vi "CBSControlling.vi"() -> ()   [LabVIEW 2015]
uses:
  classes/DataHandlerMYiTOPS.lvclass
panel:
  in  "Monitoring":T1 {"Meter" scale=0.0..20.0}
  out "appended array":string[](array[string])
  out "element":string
  out "Control-Matrix-Overview 2":i32(listbox)=-1
  in  "Controlling":T2
  in  "Cyber-physical Objects":i32(listbox)
  in  "Stop":bool
  out "Control-Matrix-Overview":i32(listbox)=-1
  # "Hard Key:"
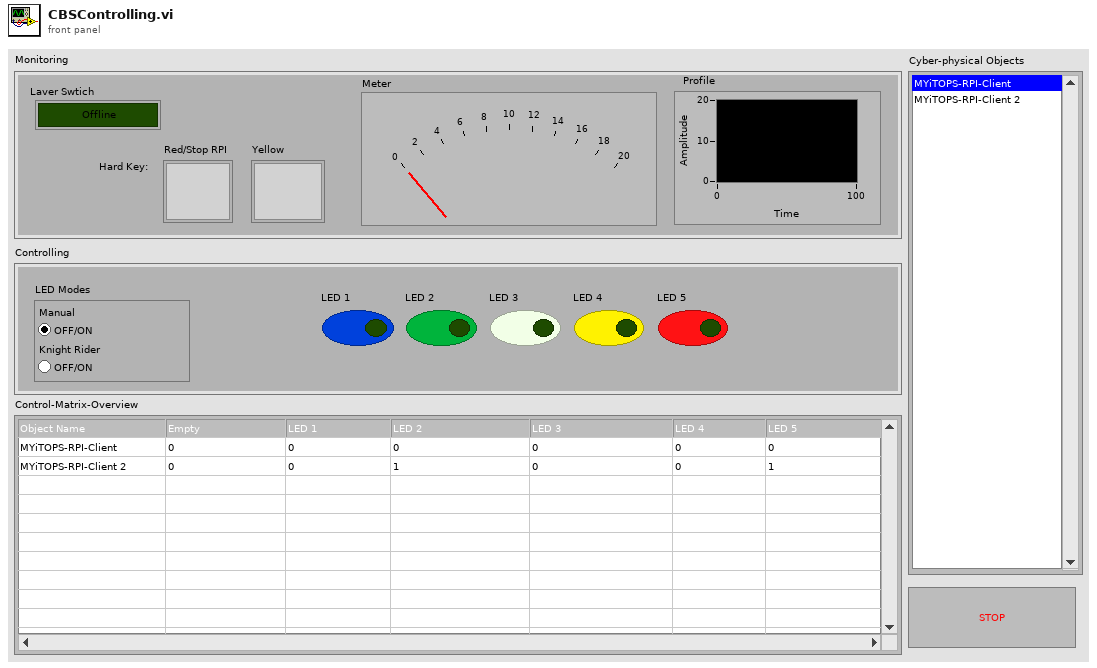
[diagram p1: front panel]
types:
  T1 = cluster{"Meter":i8, "Profile":dbl, "Yellow":bool, "Red/Stop RPI":bool, "Laver Swtich":bool}
  T2 = cluster{"LED 1":bool, "LED 5":bool, "LED 2":bool, "LED 3":bool, "LED 4":bool, "LED Modes":enum32{"Manual", "Knight Rider"}}
  T3 = enum8{"Enabled", "Disabled", "Disabled and Grayed Out"}
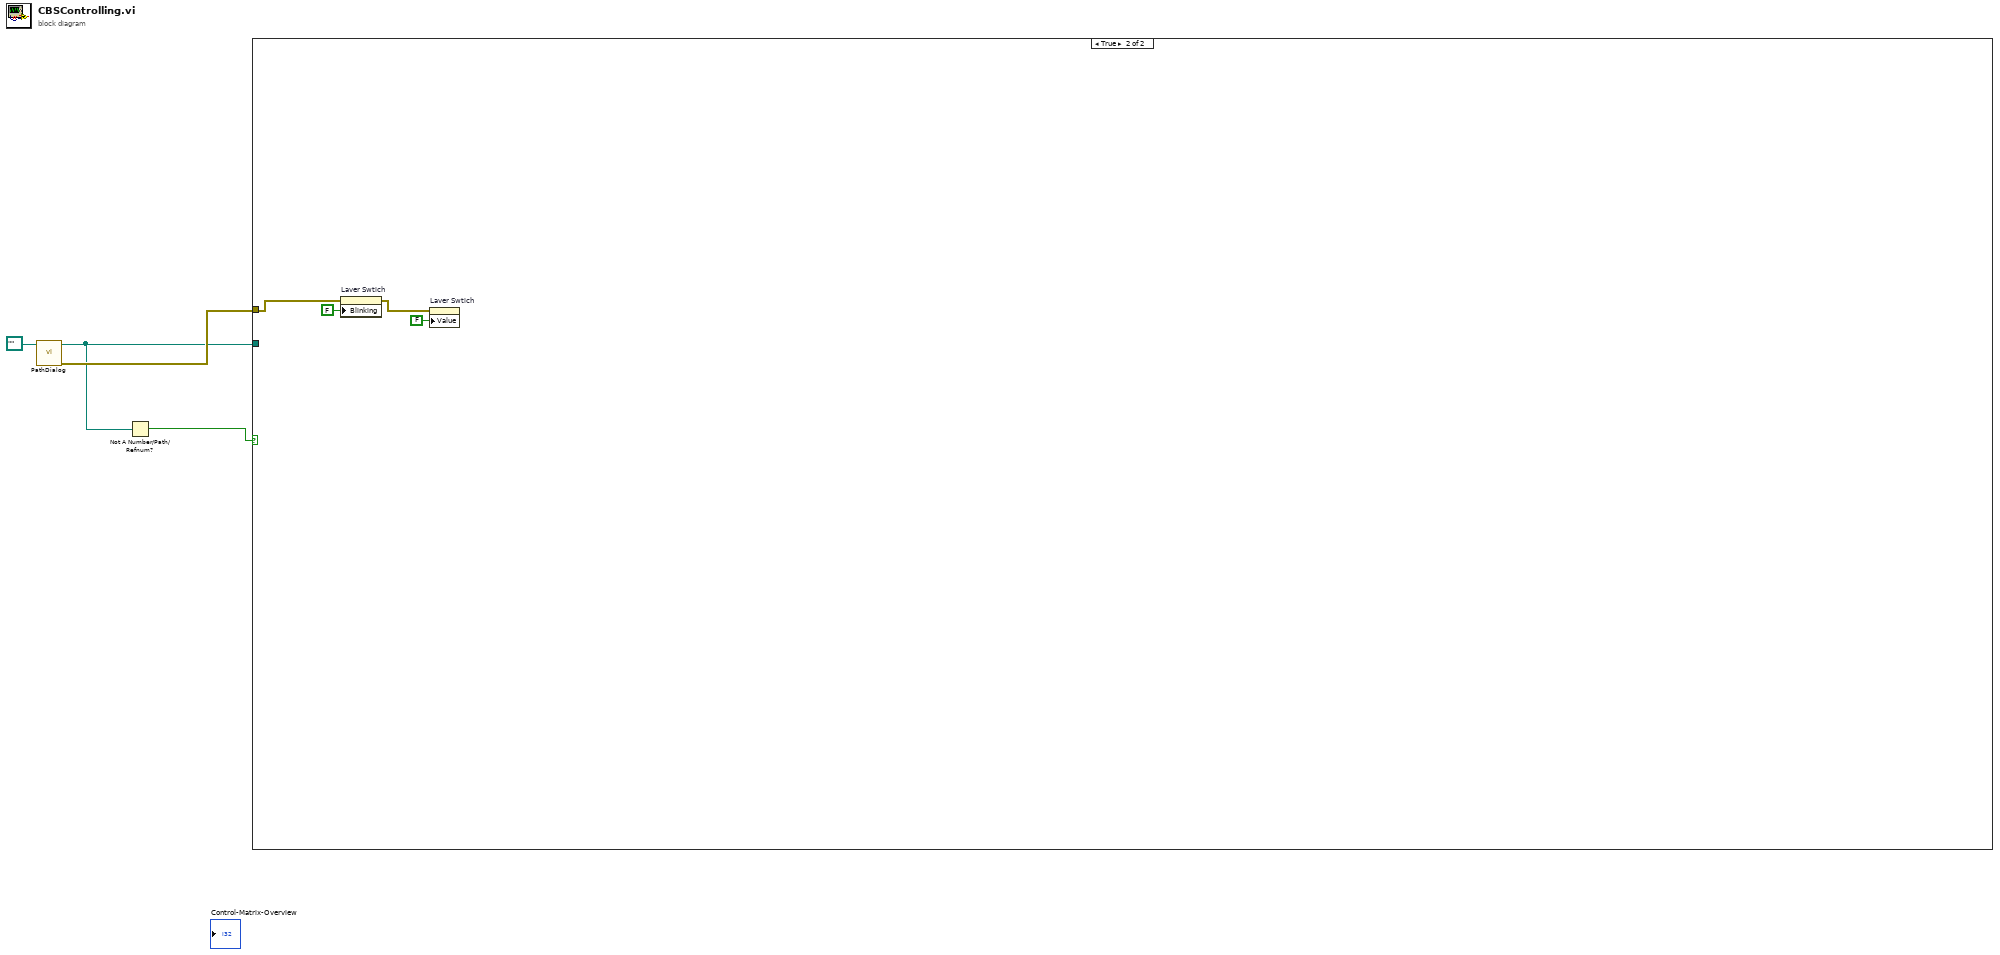
[diagram p0: block diagram]
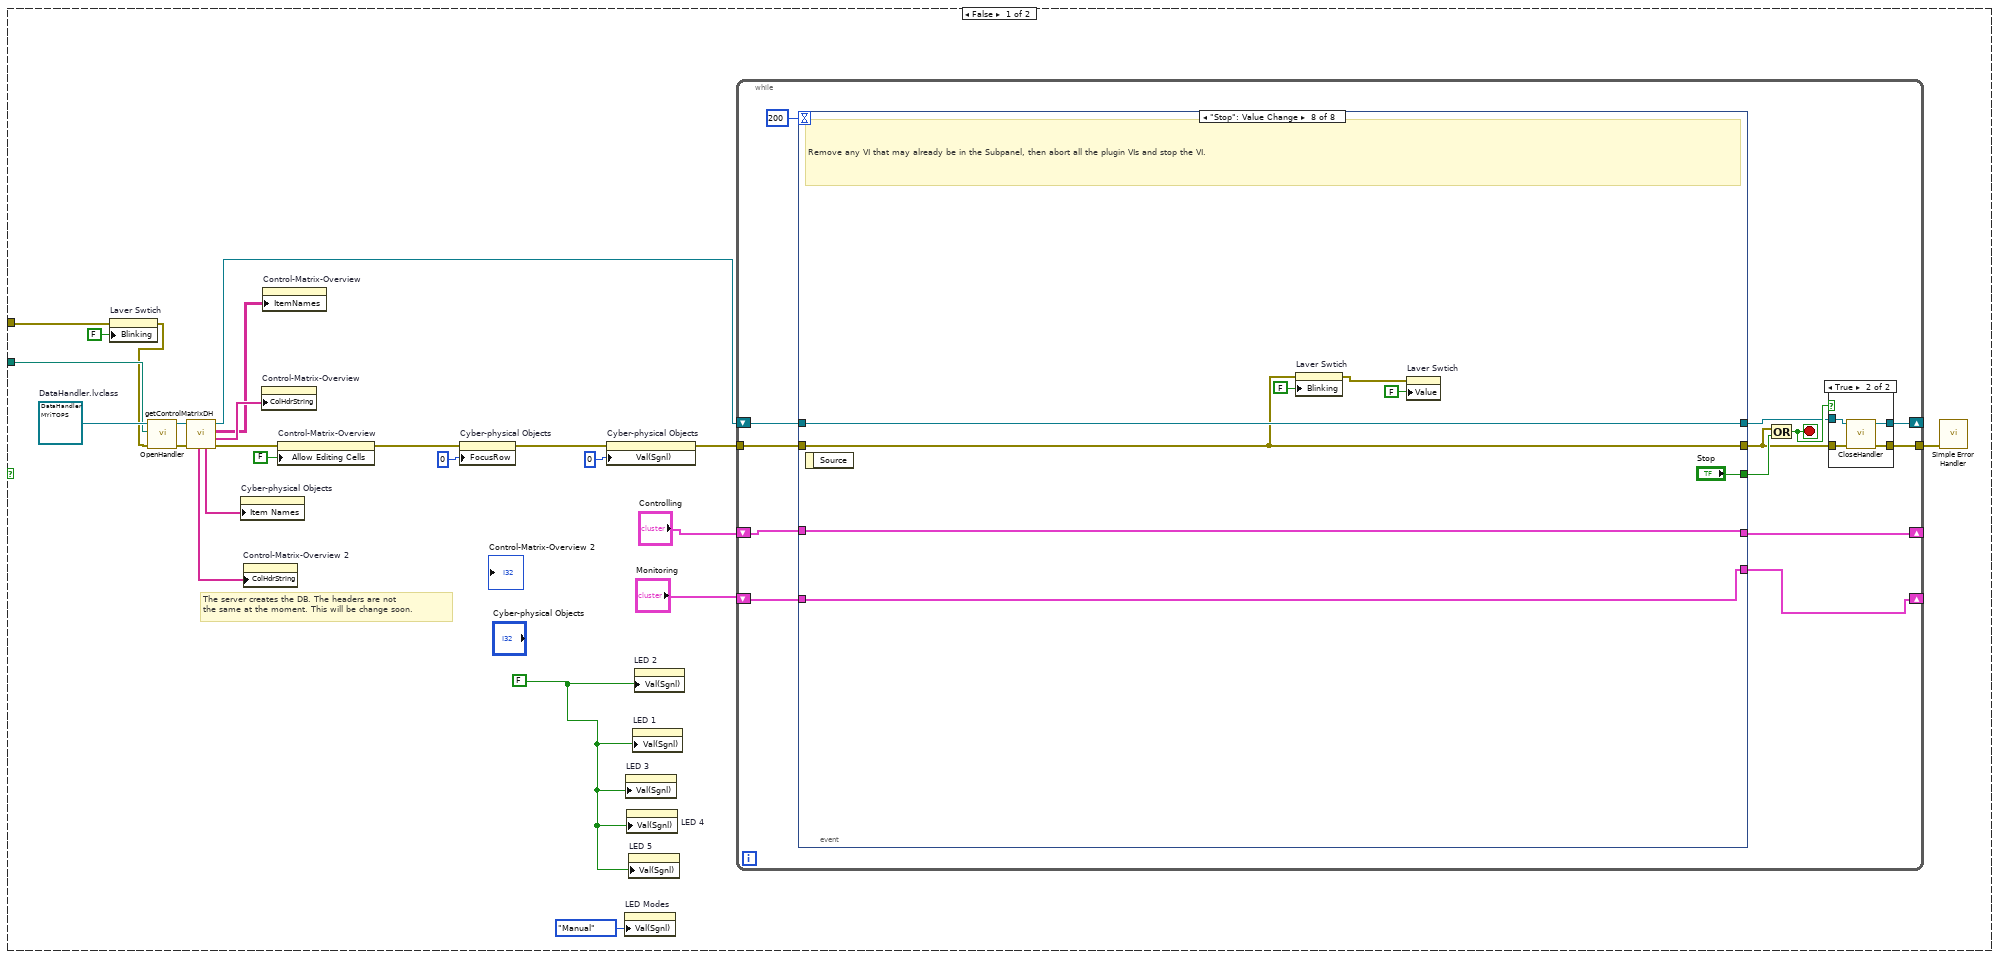
[diagram p2: hidden frame]
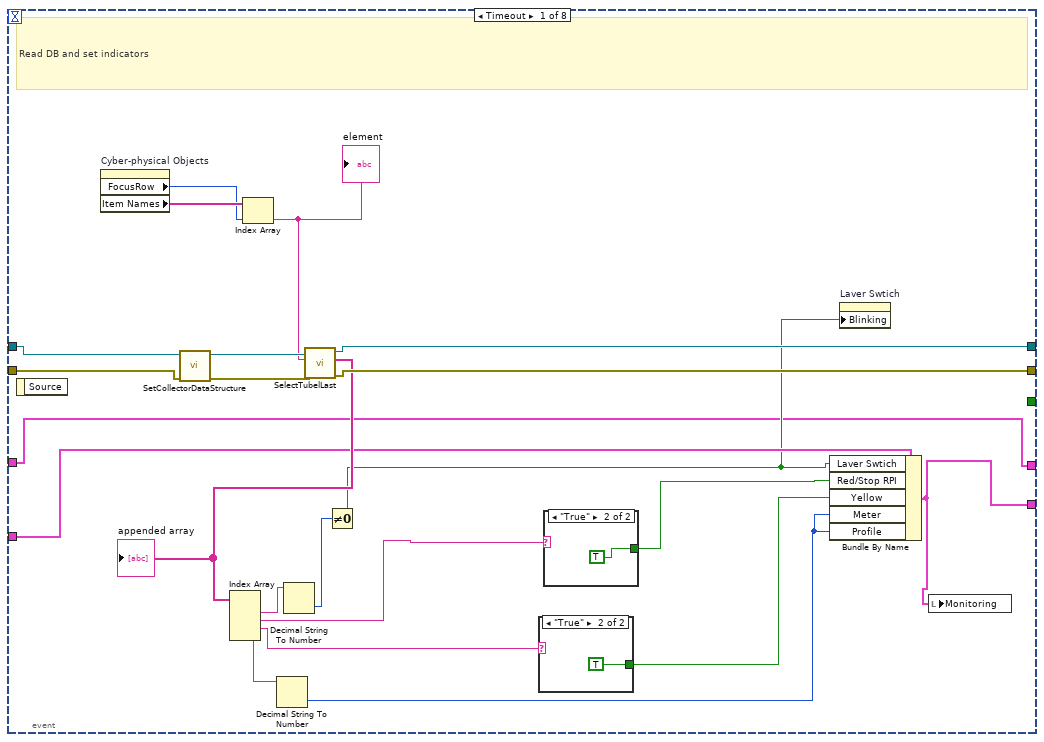
[diagram p4: hidden frame]
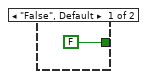
[diagram p5: hidden frame]
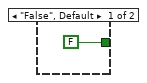
[diagram p6: hidden frame]
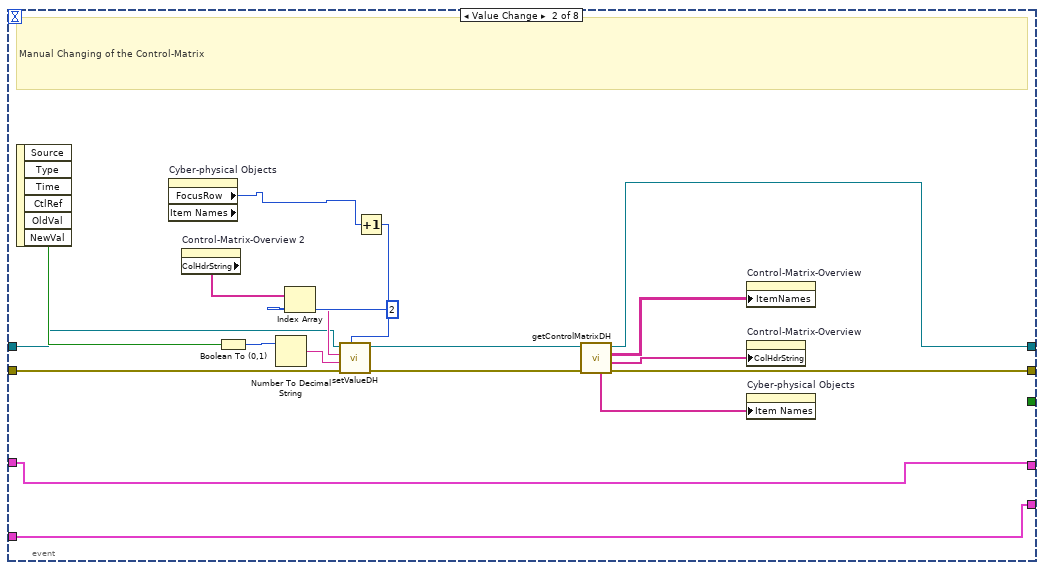
[diagram p7: hidden frame]
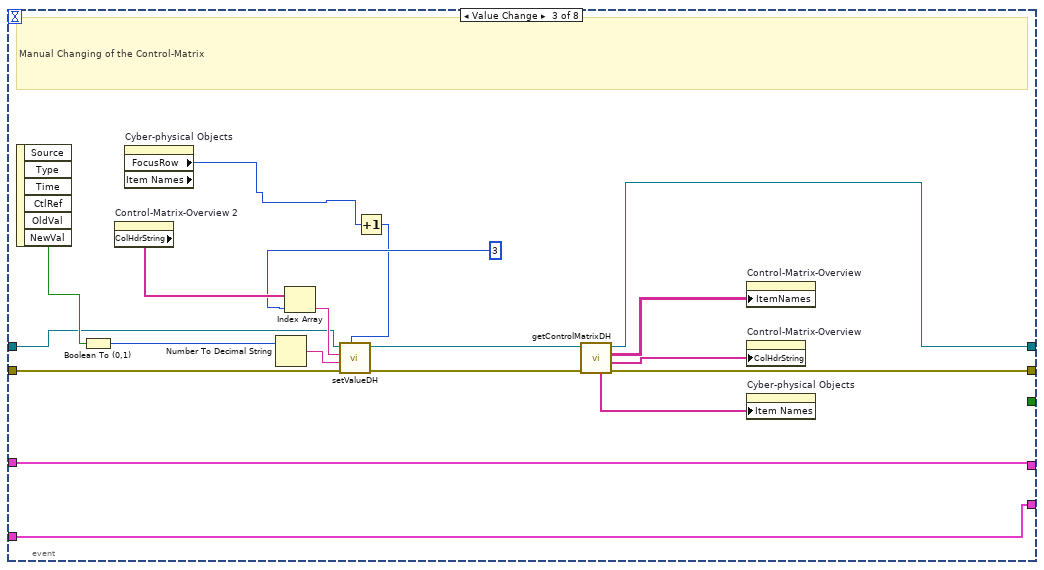
[diagram p8: hidden frame]
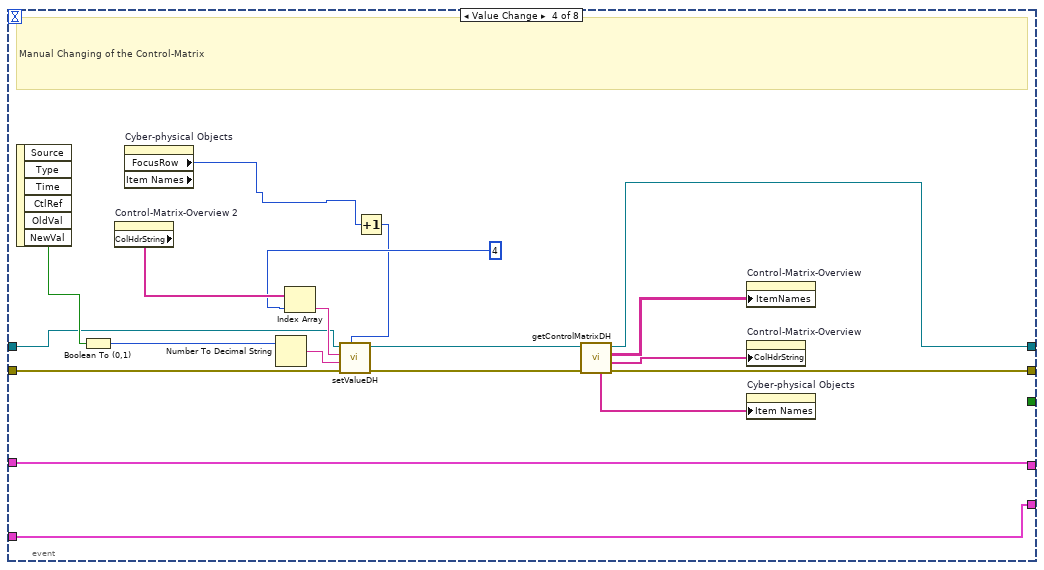
[diagram p9: hidden frame]
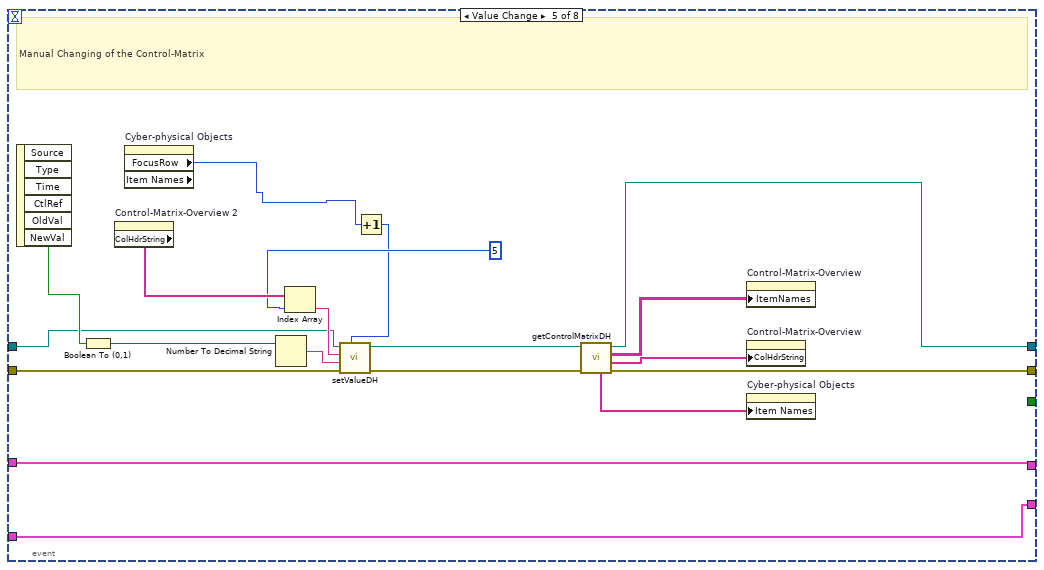
[diagram p10: hidden frame]
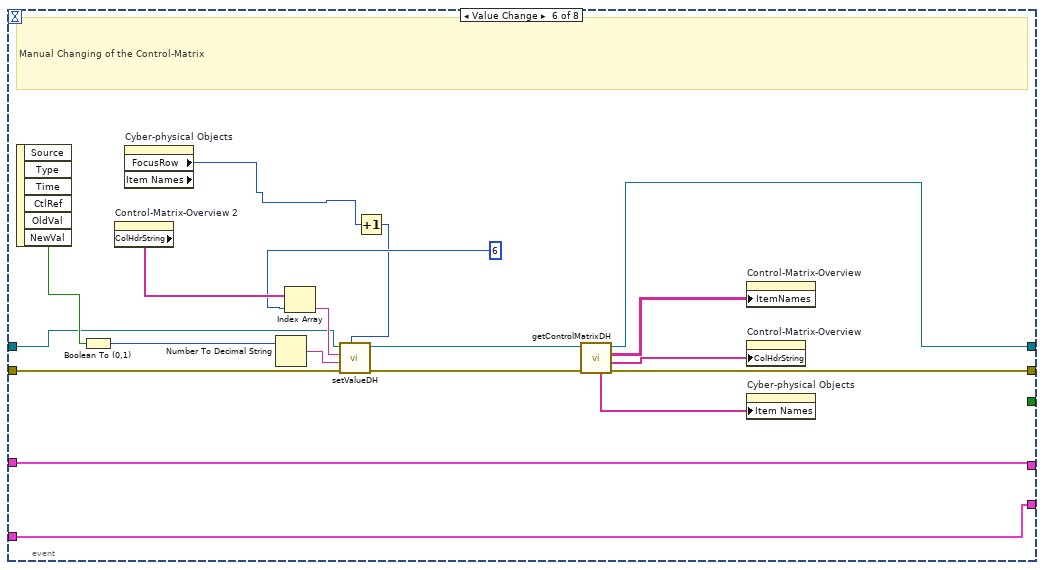
[diagram p11: hidden frame]
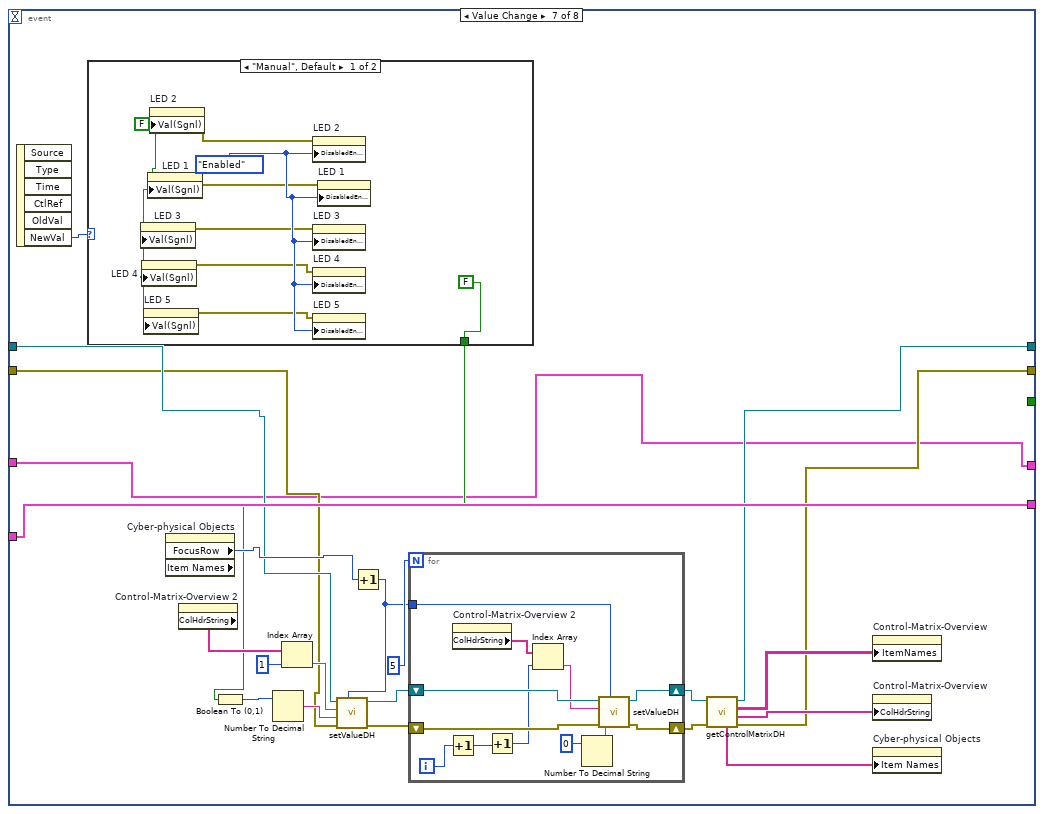
[diagram p12: hidden frame]
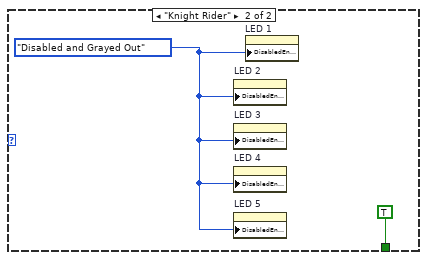
[diagram p13: hidden frame]
diagram:
  n1 = call "PathDialog.vi"("Path to Data Base in"=path "" ("Path to Data Base")) -> ("error out"=w3:errorcluster, "Path to Data Base out"=w2:path)  [unwired: 9 in]
  n2 = Not A Number/Path/Refnum?(number/path/refnum=w2) -> (NaN/Path/Refnum?=w1:bool)
  n3 = case shown="True" w1 {
    tunnel: w2 -> [w11 _]
    tunnel: w3 -> [w7 w224]
    frame False {
      w9 = FALSE ("Value")
      w24 = refnum<class "DataHandlerMYiTOPS.lvclass"> refnum  # DataHandler.lvclass
      # "The server creates the DB. The headers are not \nthe same at the moment. This will be change soon."
      n4 = property on="Laver Swtich" class="Bool (strict)"(error in=w7, "Blinking"=FALSE) -> (error out=w6:errorcluster)  [unwired: 1 in, 1 out]
      n5 = call-dynamic "OpenHandler.vi"("error in (no error)"=w6, "path to db monitoring"=w11, "DataHandling in"=w24) -> ("error out"=w23:errorcluster, "DataHandling out"=w22:refnum<class "DataHandlerMYiTOPS.lvclass">)  [unwired: 7 in]
      n6 = call-dynamic "getControlMatrixDH.vi"("error in (no error)"=w23, "DataHandler in"=w22) -> ("error out"=w20:errorcluster, "List of ColHads"=w19:string[], "Array"=w14:string[][], "DataHandler out"=w15:refnum<class "DataHandlerMYiTOPS.lvclass">, "Field Elements"=w21:string[], "List of ColHads 2"=w13:string[])  [unwired: 4 in]
      n7 = property on="Cyber-physical Objects" class="LstBox (strict)"("Item Names"=w21) -> ()  [unwired: 2 in, 2 out]
      n8 = property on="Control-Matrix-Overview 2" class="MCListbox (strict)"("ColHdrString"=w13) -> ()  [unwired: 2 in, 2 out]
      n9 = property on="Control-Matrix-Overview" class="MCListbox (strict)"("ColHdrString"=w19) -> ()  [unwired: 2 in, 2 out]
      n10 = property on="Control-Matrix-Overview" class="MCListbox (strict)"("ItemNames"=w14) -> ()  [unwired: 2 in, 2 out]
      n11 = property on="Control-Matrix-Overview" class="MCListbox (strict)"(error in=w20, "Allow Editing Cells"=FALSE) -> (error out=w16:errorcluster)  [unwired: 1 in, 1 out]
      n12 = property on="Cyber-physical Objects" class="LstBox (strict)"(error in=w16, "FocusRow"=0 ("Focus Row")) -> (error out=w17:errorcluster)  [unwired: 1 in, 1 out]
      n13 = property on="Cyber-physical Objects" class="ListBox (strict)"(error in=w17, "Val(Sgnl)"=u16 0 ("Value (Signaling)")) -> (error out=w28:errorcluster)  [unwired: 1 in, 1 out]
      n14 = property on="LED Modes" class="RadioBtnsControl (strict)"("Val(Sgnl)"=enum32{"Manual", "Knight Rider"}."Manual" ("Value (Signaling)")) -> ()  [unwired: 2 in, 2 out]
      n15 = property on="LED 3" class="Bool (strict)"("Val(Sgnl)"=w9) -> ()  [unwired: 2 in, 2 out]
      n16 = property on="LED 4" class="Bool (strict)"("Val(Sgnl)"=w9) -> ()  [unwired: 2 in, 2 out]
      n17 = property on="LED 5" class="Bool (strict)"("Val(Sgnl)"=w9) -> ()  [unwired: 2 in, 2 out]
      n18 = property on="LED 1" class="Bool (strict)"("Val(Sgnl)"=w9) -> ()  [unwired: 2 in, 2 out]
      n19 = property on="LED 2" class="Bool (strict)"("Val(Sgnl)"=w9) -> ()  [unwired: 2 in, 2 out]
      n20 = while {
        tunnel: w28 -> [w40]
        tunnel: [w35] -> w26
        shift-right: [w33] -> _
        shift-left: w15 -> [w38]
        shift-right: [w29] -> _
        shift-left: "Controlling" -> [w32]
        shift-right: [w30] -> _
        shift-left: "Monitoring" -> [w31]
        stop <- w37 stop-if-true
        n21 = event shown="[7] \"Stop\": Value Change" {
          selector: _ -> [_ _ _ _ _ _ _ _]
          dyn-events: _ -> [_ _ _ _ _ _ _ _]
          timeout: 200 -> [_ _ _ _ _ _ _ _]
          tunnel: [_ _ _ _ _ _ _ "Stop"] -> w41
          tunnel: [w62 w90 w107 w126 w145 w164 w176 w216] -> w36
          tunnel: w40 -> [w64 w92 w111 w130 w149 w168 w177 w216]
          tunnel: w38 -> [w67 w81 w98 w117 w136 w155 w179 w220]
          tunnel: [w65 w82 w99 w118 w137 w156 w178 w220] -> w34
          tunnel: w32 -> [w48 w78 w94 w113 w132 w151 w169 w219]
          tunnel: [w48 w78 w94 w113 w132 w151 w169 w219] -> w29
          tunnel: w31 -> [w52 w77 w93 w112 w131 w150 w190 w218]
          tunnel: [w51 w77 w93 w112 w131 w150 w190 w218] -> w30
          event Timeout {
            # "Read DB and set indicators"
            n22 = event-data() -> ()  [unwired: 1 in, 1 out]
            n23 = property on="Cyber-physical Objects" class="LstBox (strict)"() -> ("FocusRow"=w68:i32, "Item Names"=w69:string[])  [unwired: 2 in, 2 out]
            n24 = call-dynamic "SetCollectorDataStructure.vi"("error in (no error)"=w64, "DataHandler in"=w67) -> ("error out"=w63:errorcluster, "DataHandler out"=w66:refnum<class "DataHandlerMYiTOPS.lvclass">)  [unwired: 8 in]
            n25 = Index Array(array=w69, index=w68) -> (element=w61:string)
            "element" <- w61
            n26 = call-dynamic "SelectTubelLast.vi"("error in (no error)"=w63, "Unique Object Identifier"=w61, "DataHandler in"=w66) -> ("error out"=w62:errorcluster, "appended array"=w60:string[], "DataHandler out"=w65:refnum<class "DataHandlerMYiTOPS.lvclass">)  [unwired: 6 in]
            "appended array" <- w60
            n27 = Index Array(array=w60) -> (element #1=w59:string, element #2=w58:string, element #3=w57:string, element #4=w56:string)  [unwired: 4 in]
            n28 = Decimal String To Number(string=w56) -> (number=w55:i32)  [unwired: 2 in, 1 out]
            n29 = Decimal String To Number(string=w59) -> (number=w50:i32)  [unwired: 2 in, 1 out]
            n30 = Not Equal To 0?(x=w50) -> (x != 0?=w49:bool)
            n31 = case shown="\"True\"" w57 {
              tunnel: [FALSE TRUE] -> w54
              frame "False", Default {
              }
              frame "True" {
              }
            }
            n32 = case shown="\"True\"" w58 {
              tunnel: [FALSE TRUE] -> w53
              frame "False", Default {
              }
              frame "True" {
              }
            }
            n33 = Bundle By Name(cluster=w52, "Laver Swtich"=w49, "Red/Stop RPI"=w53, "Yellow"=w54, "Meter"=w55, "Profile"=w55) -> (w51:T1)
            n34 = property on="Laver Swtich" class="Bool (strict)"("Blinking"=w49) -> ()  [unwired: 2 in, 2 out]
            n35 = local write "Monitoring"(w51) -> ()
          }
          event "Controlling.LED 1": Value Change {
            # "Manual Changing of the Control-Matrix"
            n36 = event-data() -> ("NewVal"=w85:bool)  [unwired: 1 in, 5 out]
            n37 = property on="Cyber-physical Objects" class="LstBox (strict)" props=["FocusRow", "Item Names"]() -> ("FocusRow"=w80:i32)  [unwired: 2 in, 3 out]
            n38 = property on="Control-Matrix-Overview 2" class="MCListbox (strict)"() -> ("ColHdrString"=w88:string[])  [unwired: 2 in, 2 out]
            n39 = Boolean To (0,1)(Boolean=w85) -> (0, 1=w84:i16)
            n40 = Number To Decimal String(number=w84) -> (decimal integer string=w89:string)  [unwired: 1 in]
            n41 = Index Array(array=w88, index=2) -> (element=w86:string)
            n42 = Increment(x=w80) -> (x+1=w79:i32)
            n43 = call-dynamic "setValueDH.vi"("Focus"=w79, "error in (no error)"=w92, "Value"=w89, "ItemName"=w86, "DataHandler in"=w81) -> ("error out"=w91:errorcluster, "DataHandler out"=w83:refnum<class "DataHandlerMYiTOPS.lvclass">)  [unwired: 5 in]
            n44 = call-dynamic "getControlMatrixDH.vi"("error in (no error)"=w91, "DataHandler in"=w83) -> ("error out"=w90:errorcluster, "List of ColHads"=w75:string[], "Array"=w74:string[][], "DataHandler out"=w82:refnum<class "DataHandlerMYiTOPS.lvclass">, "Field Elements"=w76:string[])  [unwired: 4 in, 1 out]
            n45 = property on="Control-Matrix-Overview" class="MCListbox (strict)"("ItemNames"=w74) -> ()  [unwired: 2 in, 2 out]
            n46 = property on="Control-Matrix-Overview" class="MCListbox (strict)"("ColHdrString"=w75) -> ()  [unwired: 2 in, 2 out]
            n47 = property on="Cyber-physical Objects" class="LstBox (strict)"("Item Names"=w76) -> ()  [unwired: 2 in, 2 out]
          }
          event "Controlling.LED 2": Value Change {
            # "Manual Changing of the Control-Matrix"
            n48 = event-data() -> ("NewVal"=w102:bool)  [unwired: 1 in, 5 out]
            n49 = Boolean To (0,1)(Boolean=w102) -> (0, 1=w101:i16)
            n50 = property on="Control-Matrix-Overview 2" class="MCListbox (strict)"() -> ("ColHdrString"=w105:string[])  [unwired: 2 in, 2 out]
            n51 = property on="Cyber-physical Objects" class="LstBox (strict)" props=["FocusRow", "Item Names"]() -> ("FocusRow"=w96:i32)  [unwired: 2 in, 3 out]
            n52 = Number To Decimal String(number=w101) -> (decimal integer string=w106:string)  [unwired: 1 in]
            n53 = Index Array(array=w105, index=3) -> (element=w103:string)
            n54 = Increment(x=w96) -> (x+1=w95:i32)
            n55 = call-dynamic "setValueDH.vi"("Focus"=w95, "error in (no error)"=w111, "Value"=w106, "ItemName"=w103, "DataHandler in"=w98) -> ("error out"=w108:errorcluster, "DataHandler out"=w100:refnum<class "DataHandlerMYiTOPS.lvclass">)  [unwired: 5 in]
            n56 = call-dynamic "getControlMatrixDH.vi"("error in (no error)"=w108, "DataHandler in"=w100) -> ("error out"=w107:errorcluster, "List of ColHads"=w109:string[], "Array"=w97:string[][], "DataHandler out"=w99:refnum<class "DataHandlerMYiTOPS.lvclass">, "Field Elements"=w110:string[])  [unwired: 4 in, 1 out]
            n57 = property on="Control-Matrix-Overview" class="MCListbox (strict)"("ItemNames"=w97) -> ()  [unwired: 2 in, 2 out]
            n58 = property on="Control-Matrix-Overview" class="MCListbox (strict)"("ColHdrString"=w109) -> ()  [unwired: 2 in, 2 out]
            n59 = property on="Cyber-physical Objects" class="LstBox (strict)"("Item Names"=w110) -> ()  [unwired: 2 in, 2 out]
          }
          event "Controlling.LED 3": Value Change {
            # "Manual Changing of the Control-Matrix"
            n60 = event-data() -> ("NewVal"=w121:bool)  [unwired: 1 in, 5 out]
            n61 = Boolean To (0,1)(Boolean=w121) -> (0, 1=w120:i16)
            n62 = property on="Control-Matrix-Overview 2" class="MCListbox (strict)"() -> ("ColHdrString"=w124:string[])  [unwired: 2 in, 2 out]
            n63 = property on="Cyber-physical Objects" class="LstBox (strict)" props=["FocusRow", "Item Names"]() -> ("FocusRow"=w115:i32)  [unwired: 2 in, 3 out]
            n64 = Number To Decimal String(number=w120) -> (decimal integer string=w125:string)  [unwired: 1 in]
            n65 = Index Array(array=w124, index=4) -> (element=w122:string)
            n66 = Increment(x=w115) -> (x+1=w114:i32)
            n67 = call-dynamic "setValueDH.vi"("Focus"=w114, "error in (no error)"=w130, "Value"=w125, "ItemName"=w122, "DataHandler in"=w117) -> ("error out"=w127:errorcluster, "DataHandler out"=w119:refnum<class "DataHandlerMYiTOPS.lvclass">)  [unwired: 5 in]
            n68 = call-dynamic "getControlMatrixDH.vi"("error in (no error)"=w127, "DataHandler in"=w119) -> ("error out"=w126:errorcluster, "List of ColHads"=w128:string[], "Array"=w116:string[][], "DataHandler out"=w118:refnum<class "DataHandlerMYiTOPS.lvclass">, "Field Elements"=w129:string[])  [unwired: 4 in, 1 out]
            n69 = property on="Control-Matrix-Overview" class="MCListbox (strict)"("ItemNames"=w116) -> ()  [unwired: 2 in, 2 out]
            n70 = property on="Control-Matrix-Overview" class="MCListbox (strict)"("ColHdrString"=w128) -> ()  [unwired: 2 in, 2 out]
            n71 = property on="Cyber-physical Objects" class="LstBox (strict)"("Item Names"=w129) -> ()  [unwired: 2 in, 2 out]
          }
          event "Controlling.LED 4": Value Change {
            # "Manual Changing of the Control-Matrix"
            n72 = event-data() -> ("NewVal"=w140:bool)  [unwired: 1 in, 5 out]
            n73 = Boolean To (0,1)(Boolean=w140) -> (0, 1=w139:i16)
            n74 = property on="Control-Matrix-Overview 2" class="MCListbox (strict)"() -> ("ColHdrString"=w143:string[])  [unwired: 2 in, 2 out]
            n75 = property on="Cyber-physical Objects" class="LstBox (strict)" props=["FocusRow", "Item Names"]() -> ("FocusRow"=w134:i32)  [unwired: 2 in, 3 out]
            n76 = Number To Decimal String(number=w139) -> (decimal integer string=w144:string)  [unwired: 1 in]
            n77 = Index Array(array=w143, index=5) -> (element=w141:string)
            n78 = Increment(x=w134) -> (x+1=w133:i32)
            n79 = call-dynamic "setValueDH.vi"("Focus"=w133, "error in (no error)"=w149, "Value"=w144, "ItemName"=w141, "DataHandler in"=w136) -> ("error out"=w146:errorcluster, "DataHandler out"=w138:refnum<class "DataHandlerMYiTOPS.lvclass">)  [unwired: 5 in]
            n80 = call-dynamic "getControlMatrixDH.vi"("error in (no error)"=w146, "DataHandler in"=w138) -> ("error out"=w145:errorcluster, "List of ColHads"=w147:string[], "Array"=w135:string[][], "DataHandler out"=w137:refnum<class "DataHandlerMYiTOPS.lvclass">, "Field Elements"=w148:string[])  [unwired: 4 in, 1 out]
            n81 = property on="Control-Matrix-Overview" class="MCListbox (strict)"("ItemNames"=w135) -> ()  [unwired: 2 in, 2 out]
            n82 = property on="Control-Matrix-Overview" class="MCListbox (strict)"("ColHdrString"=w147) -> ()  [unwired: 2 in, 2 out]
            n83 = property on="Cyber-physical Objects" class="LstBox (strict)"("Item Names"=w148) -> ()  [unwired: 2 in, 2 out]
          }
          event "Controlling.LED 5": Value Change {
            # "Manual Changing of the Control-Matrix"
            n84 = event-data() -> ("NewVal"=w159:bool)  [unwired: 1 in, 5 out]
            n85 = Boolean To (0,1)(Boolean=w159) -> (0, 1=w158:i16)
            n86 = property on="Control-Matrix-Overview 2" class="MCListbox (strict)"() -> ("ColHdrString"=w162:string[])  [unwired: 2 in, 2 out]
            n87 = property on="Cyber-physical Objects" class="LstBox (strict)" props=["FocusRow", "Item Names"]() -> ("FocusRow"=w153:i32)  [unwired: 2 in, 3 out]
            n88 = Number To Decimal String(number=w158) -> (decimal integer string=w163:string)  [unwired: 1 in]
            n89 = Index Array(array=w162, index=6) -> (element=w160:string)
            n90 = Increment(x=w153) -> (x+1=w152:i32)
            n91 = call-dynamic "setValueDH.vi"("Focus"=w152, "error in (no error)"=w168, "Value"=w163, "ItemName"=w160, "DataHandler in"=w155) -> ("error out"=w165:errorcluster, "DataHandler out"=w157:refnum<class "DataHandlerMYiTOPS.lvclass">)  [unwired: 5 in]
            n92 = call-dynamic "getControlMatrixDH.vi"("error in (no error)"=w165, "DataHandler in"=w157) -> ("error out"=w164:errorcluster, "List of ColHads"=w166:string[], "Array"=w154:string[][], "DataHandler out"=w156:refnum<class "DataHandlerMYiTOPS.lvclass">, "Field Elements"=w167:string[])  [unwired: 4 in, 1 out]
            n93 = property on="Control-Matrix-Overview" class="MCListbox (strict)"("ItemNames"=w154) -> ()  [unwired: 2 in, 2 out]
            n94 = property on="Control-Matrix-Overview" class="MCListbox (strict)"("ColHdrString"=w166) -> ()  [unwired: 2 in, 2 out]
            n95 = property on="Cyber-physical Objects" class="LstBox (strict)"("Item Names"=w167) -> ()  [unwired: 2 in, 2 out]
          }
          event "Controlling.LED Modes": Value Change {
            n96 = event-data() -> ("NewVal"=w191:enum32{"Manual", "Knight Rider"})  [unwired: 1 in, 5 out]
            n97 = case shown="\"Manual\", Default" w191 {
              tunnel: [FALSE TRUE] -> w180
              frame "Manual", Default {
                w208 = FALSE ("Value")
                w211 = T3."Enabled" ("Disabled")
                n98 = property on="LED 3" class="Bool (strict)"("Val(Sgnl)"=w208) -> (error out=w206:errorcluster)  [unwired: 2 in, 1 out]
                n99 = property on="LED 4" class="Bool (strict)"("Val(Sgnl)"=w208) -> (error out=w205:errorcluster)  [unwired: 2 in, 1 out]
                n100 = property on="LED 5" class="Bool (strict)"("Val(Sgnl)"=w208) -> (error out=w204:errorcluster)  [unwired: 2 in, 1 out]
                n101 = property on="LED 1" class="Bool (strict)"("Val(Sgnl)"=w208) -> (error out=w207:errorcluster)  [unwired: 2 in, 1 out]
                n102 = property on="LED 2" class="Bool (strict)"("Val(Sgnl)"=w208) -> (error out=w209:errorcluster)  [unwired: 2 in, 1 out]
                n103 = property on="LED 2" class="Bool (strict)"(error in=w209, "DisabledEnum"=w211) -> ()  [unwired: 1 in, 2 out]
                n104 = property on="LED 3" class="Bool (strict)"(error in=w206, "DisabledEnum"=w211) -> ()  [unwired: 1 in, 2 out]
                n105 = property on="LED 4" class="Bool (strict)"(error in=w205, "DisabledEnum"=w211) -> ()  [unwired: 1 in, 2 out]
                n106 = property on="LED 5" class="Bool (strict)"(error in=w204, "DisabledEnum"=w211) -> ()  [unwired: 1 in, 2 out]
                n107 = property on="LED 1" class="Bool (strict)"(error in=w207, "DisabledEnum"=w211) -> ()  [unwired: 1 in, 2 out]
              }
              frame "Knight Rider" {
                w213 = T3."Disabled and Grayed Out" ("Disabled")
                n108 = property on="LED 2" class="Bool (strict)"("DisabledEnum"=w213) -> ()  [unwired: 2 in, 2 out]
                n109 = property on="LED 3" class="Bool (strict)"("DisabledEnum"=w213) -> ()  [unwired: 2 in, 2 out]
                n110 = property on="LED 4" class="Bool (strict)"("DisabledEnum"=w213) -> ()  [unwired: 2 in, 2 out]
                n111 = property on="LED 5" class="Bool (strict)"("DisabledEnum"=w213) -> ()  [unwired: 2 in, 2 out]
                n112 = property on="LED 1" class="Bool (strict)"("DisabledEnum"=w213) -> ()  [unwired: 2 in, 2 out]
              }
            }
            n113 = property on="Cyber-physical Objects" class="LstBox (strict)" props=["FocusRow", "Item Names"]() -> ("FocusRow"=w185:i32)  [unwired: 2 in, 3 out]
            n114 = property on="Control-Matrix-Overview 2" class="MCListbox (strict)"() -> ("ColHdrString"=w188:string[])  [unwired: 2 in, 2 out]
            n115 = Boolean To (0,1)(Boolean=w180) -> (0, 1=w186:i16)
            n116 = Number To Decimal String(number=w186) -> (decimal integer string=w189:string)  [unwired: 1 in]
            n117 = Index Array(array=w188, index=1) -> (element=w187:string)
            n118 = Increment(x=w185) -> (x+1=w170:i32)
            n119 = call-dynamic "setValueDH.vi"("Focus"=w170, "error in (no error)"=w177, "Value"=w189, "ItemName"=w187, "DataHandler in"=w179) -> ("error out"=w175:errorcluster, "DataHandler out"=w173:refnum<class "DataHandlerMYiTOPS.lvclass">)  [unwired: 5 in]
            n120 = for {
              N: 5 -> [_]
              shift-right: [w202] -> w174
              shift-left: w175 -> [w203]
              shift-right: [w200] -> w172
              shift-left: w173 -> [w201]
              tunnel: w170 -> [w193]
              i -> [w198]
              n121 = Increment(x=w198) -> (x+1=w197:i32)
              n122 = property on="Control-Matrix-Overview 2" class="MCListbox (strict)"() -> ("ColHdrString"=w196:string[])  [unwired: 2 in, 2 out]
              n123 = Increment(x=w197) -> (x+1=w195:i32)
              n124 = Index Array(array=w196, index=w195) -> (element=w194:string)
              n125 = Number To Decimal String(number=0) -> (decimal integer string=w199:string)  [unwired: 1 in]
              n126 = call-dynamic "setValueDH.vi"("Focus"=w193, "error in (no error)"=w203, "Value"=w199, "ItemName"=w194, "DataHandler in"=w201) -> ("error out"=w202:errorcluster, "DataHandler out"=w200:refnum<class "DataHandlerMYiTOPS.lvclass">)  [unwired: 5 in]
            }
            n127 = call-dynamic "getControlMatrixDH.vi"("error in (no error)"=w174, "DataHandler in"=w172) -> ("error out"=w176:errorcluster, "List of ColHads"=w183:string[], "Array"=w182:string[][], "DataHandler out"=w178:refnum<class "DataHandlerMYiTOPS.lvclass">, "Field Elements"=w184:string[])  [unwired: 4 in, 1 out]
            n128 = property on="Control-Matrix-Overview" class="MCListbox (strict)"("ItemNames"=w182) -> ()  [unwired: 2 in, 2 out]
            n129 = property on="Control-Matrix-Overview" class="MCListbox (strict)"("ColHdrString"=w183) -> ()  [unwired: 2 in, 2 out]
            n130 = property on="Cyber-physical Objects" class="LstBox (strict)"("Item Names"=w184) -> ()  [unwired: 2 in, 2 out]
          }
          event "Stop": Value Change {
            # "Remove any VI that may already be in the Subpanel, then abort all the plugin VIs and stop the VI."
            n131 = event-data() -> ()  [unwired: 1 in, 1 out]
            n132 = property on="Laver Swtich" class="Bool (strict)"(error in=w216, "Blinking"=FALSE) -> (error out=w215:errorcluster)  [unwired: 1 in, 1 out]
            n133 = property on="Laver Swtich" class="Bool (strict)"(error in=w215, "Value"=FALSE) -> ()  [unwired: 1 in, 2 out]
          }
        }
        n134 = Or(x=w36, y=w41) -> (x .or. y?=w37:bool)
        n135 = case shown="True" w37 {
          tunnel: w36 -> [w43 w46]
          tunnel: [w43 w47] -> w35
          tunnel: w34 -> [w42 w45]
          tunnel: [w42 w44] -> w33
          frame False {
          }
          frame True {
            n136 = call-dynamic "CloseHandler.vi"("error in (no error)"=w46, "DataHandling in"=w45) -> ("error out"=w47:errorcluster, "DataHandling out"=w44:refnum<class "DataHandlerMYiTOPS.lvclass">)  [unwired: 8 in]
          }
        }
      }
      n137 = call <vilib>:"Simple Error Handler.vi"("error in (no error)"=w26) -> ()  [unwired: 4 in, 5 out]
    }
    frame True {
      n138 = property on="Laver Swtich" class="Bool (strict)"(error in=w224, "Blinking"=FALSE) -> (error out=w222:errorcluster)  [unwired: 1 in, 1 out]
      n139 = property on="Laver Swtich" class="Bool (strict)"(error in=w222, "Value"=FALSE) -> ()  [unwired: 1 in, 2 out]
    }
  }
